vi "pierwiastki_zespolone.vi"(9 "delta":dbl, 10 "bp":dbl, 11 "ap":dbl) -> (2 "x2":cdb, 3 "x1":cdb)   [LabVIEW 2020]
doc: "Obliczanie zespolonych pierwiastków wielomianu 2 stopnia"
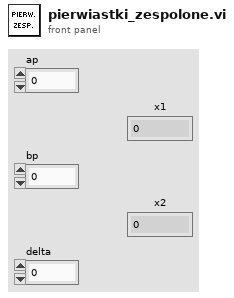
[diagram p1: front panel]
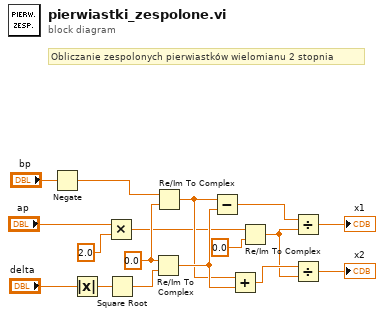
[diagram p0: block diagram]
diagram:
  w10 = 0.0 ("x")
  # "Obliczanie zespolonych pierwiastków wielomianu 2 stopnia"
  n1 = Negate(x="bp") -> (-x=w1:dbl)
  n2 = Absolute Value(x="delta") -> (abs(x)=w17:dbl)
  n3 = Multiply(x="ap", y=2.0) -> (x*y=w4:dbl)
  n4 = Square Root(x=w17) -> (sqrt(x)=w5:dbl)
  n5 = Re/Im To Complex(1:w5, 2:w10) -> (0:w13:cdb)
  n6 = Re/Im To Complex(1:w10, 2:w1) -> (0:w12:cdb)
  n7 = Subtract(x=w12, y=w13) -> (x-y=w9:cdb)
  n8 = Add(x=w12, y=w13) -> (x+y=w14:cdb)
  n9 = Re/Im To Complex(1:0.0 ("y"), 2:w4) -> (0:w3:cdb)
  n10 = Divide(x=w9, y=w3) -> (x/y=→"x1":cdb)
  n11 = Divide(x=w14, y=w3) -> (x/y=→"x2":cdb)
